vi "DeviceSelect.vi"() -> ()   [LabVIEW 2020]
uses:
  GlobalDeviceList.vi
panel:
  out "通道数量":string
  in  "全选按钮":T1
  in  "通道状态":cluster{"通道0":T2, "通道1":T2, "通道2":T2, "通道3":T2}
  out "勾选的设备":string[](array[string])
  in  "取消":T3
  in  "确定":T4
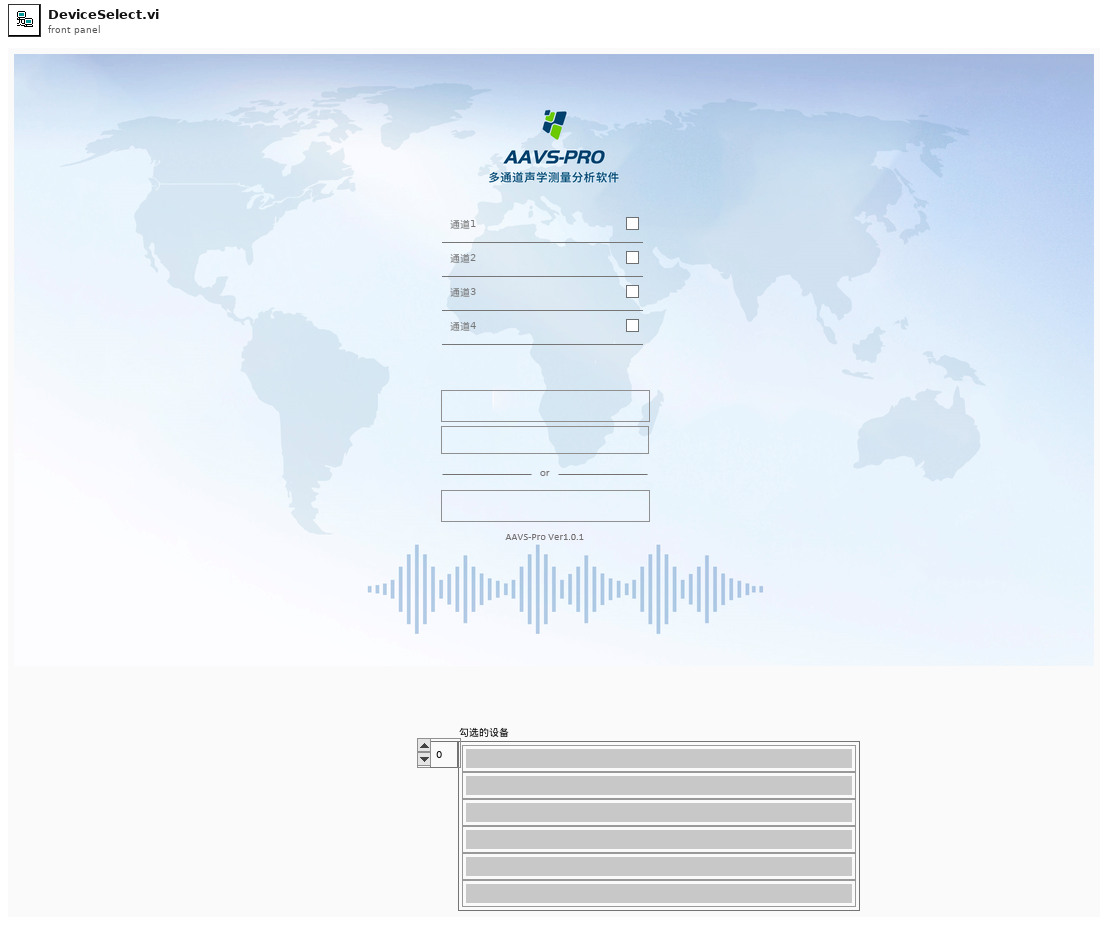
[diagram p1: front panel]
types:
  T1 = typedef "首页全选按钮.ctl" = bool
  T2 = typedef "首页复选框.ctl" = bool
  T3 = typedef "首页取消按钮.ctl" = bool
  T4 = typedef "首页确认按钮.ctl" = bool
  T5 = cluster{"通道0":bool, "通道1":bool, "通道2":bool, "通道3":bool}
  T6 = cluster{"勾选的设备":refnum<visa-resource-name>[], "设备启用状态":cluster{"通道0":bool, "通道1":bool, "通道2":bool, "通道3":bool}}
  T7 = enum32{"Invalid", "Standard", "Closed", "Hidden", "Minimized", "Maximized"}
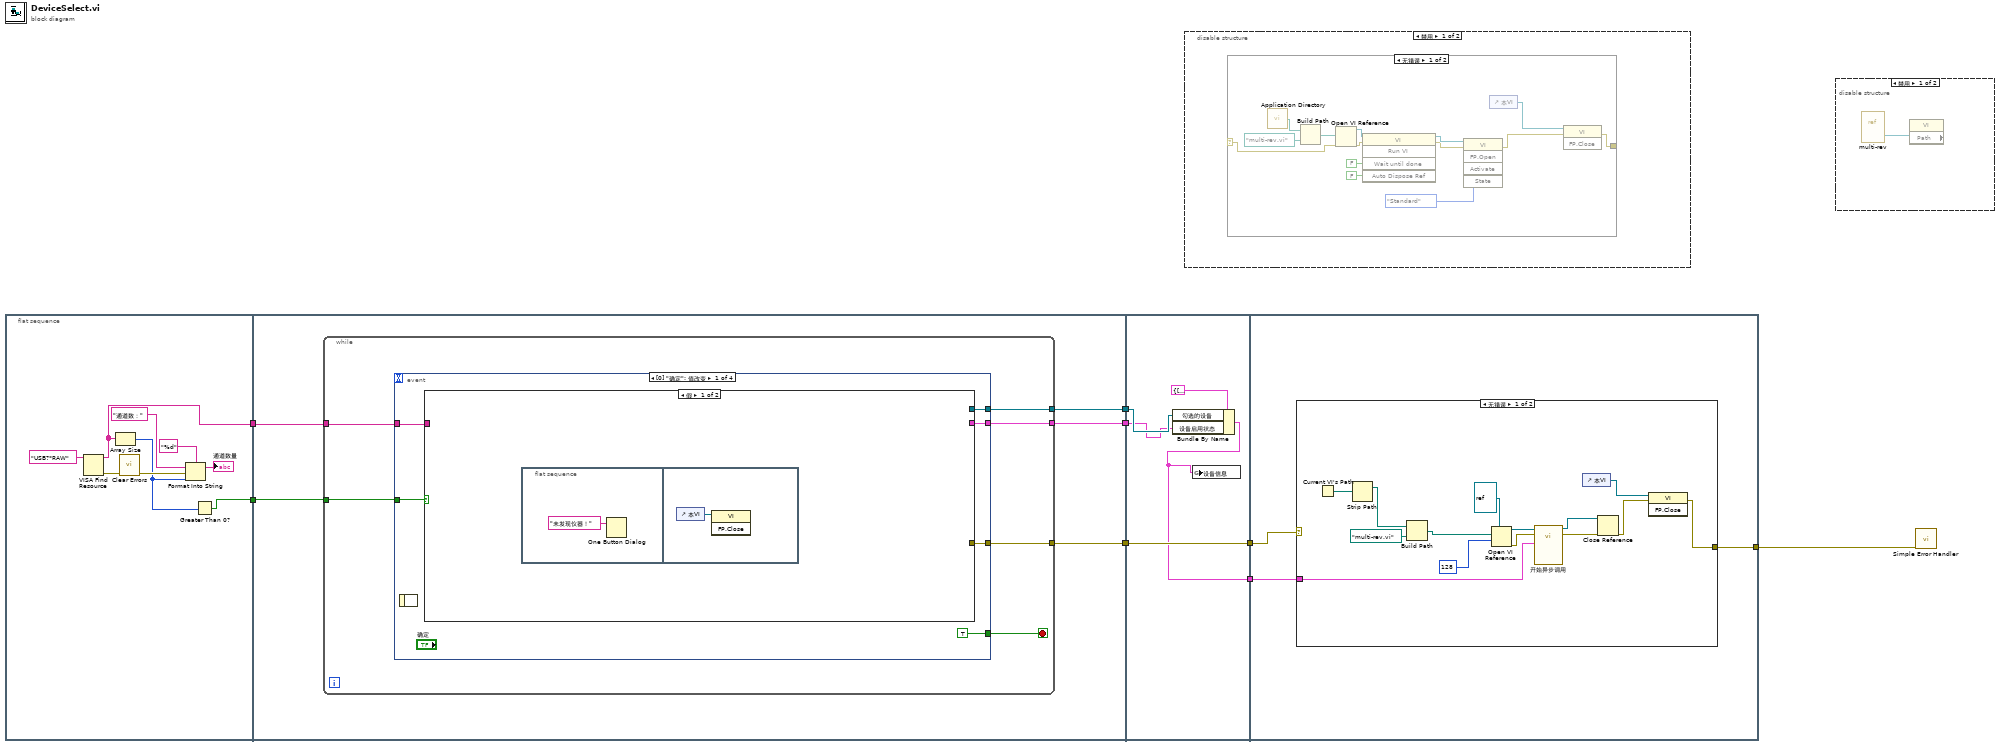
[diagram p0: block diagram]
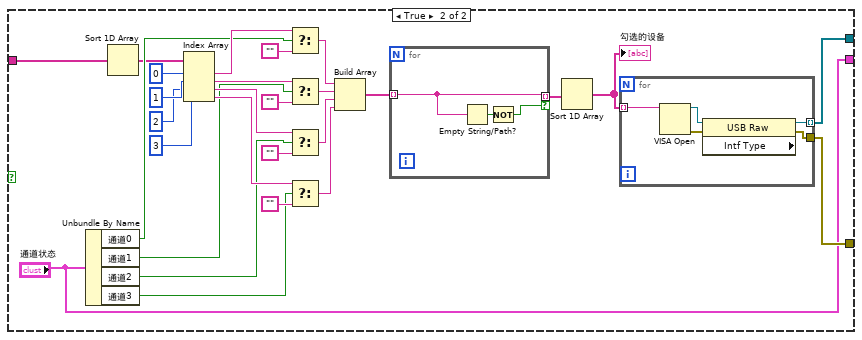
[diagram p5: hidden frame]
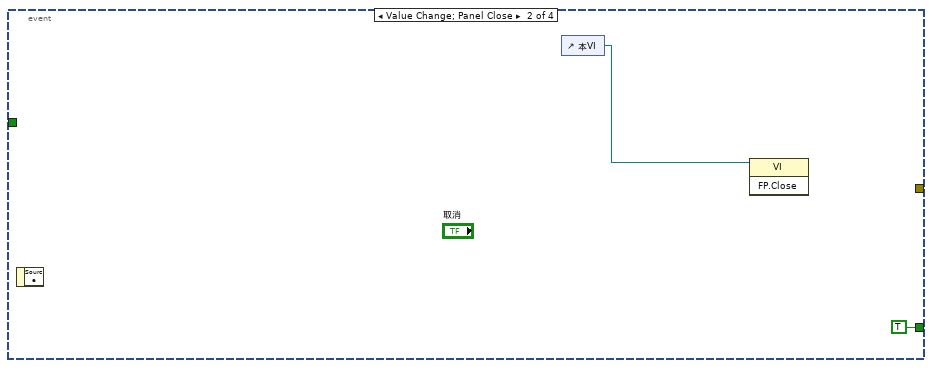
[diagram p6: hidden frame]
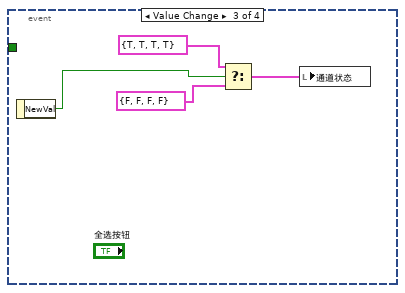
[diagram p7: hidden frame]
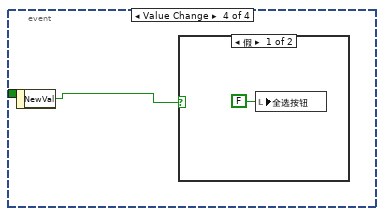
[diagram p8: hidden frame]
diagram:
  n1 = flat-sequence {
    tunnel: [w16] -> w2
    tunnel: [w9] -> w1
    tunnel: [w22] -> w7
    tunnel: [w21] -> w6
    tunnel: [w20] -> w4
    tunnel: w2 -> [w19]
    tunnel: w1 -> [w18]
    tunnel: w7 -> [w83]
    tunnel: w6 -> [w85]
    tunnel: [w85] -> w5
    tunnel: w4 -> [w82]
    tunnel: [w81] -> w3
    tunnel: [w86] -> w8
    tunnel: w5 -> [w88]
    tunnel: w3 -> [w87]
    frame #0 {
      n2 = VISA Find Resource(11:"USB?*RAW" ("表达式(\"?*\")")) -> (0:w12:errorcluster, 3:w16:string[])  [unwired: 2 in, 1 out]
      n3 = Array Size(array=w16) -> (size(s)=w10:i32)
      n4 = call <vilib>:"Clear Errors.vi"("error in (no error)"=w12) -> ("error out"=w11:errorcluster)  [unwired: 5 in, 1 out]
      n5 = Format Into String(format string="%d" ("格式字符串"), initial string="通道数：" ("初始字符串"), error in=w11, w10) -> (resulting string=→"通道数量":string)  [unwired: 1 out]
      n6 = Greater Than 0?(x=w10) -> (x > 0?=w9:bool)
    }
    frame #1 {
      n7 = while {
        tunnel: [w28] -> w22
        tunnel: [w27] -> w21
        tunnel: [w26] -> w20
        tunnel: w19 -> [w25]
        tunnel: w18 -> [w23]
        stop <- w24 stop-if-true
        n8 = event shown="[0] \"确定\": 值改变" {
          selector: _ -> [_ _ _ _]
          dyn-events: _ -> [_ _ _ _]
          timeout: _ -> [_ _ _ _]
          tunnel: [w34 _ _ _] -> w28
          tunnel: [w33 _ _ _] -> w27
          tunnel: [w31 _ _ _] -> w26
          tunnel: w25 -> [w32 _ _ _]
          tunnel: [TRUE TRUE _ _] -> w24
          tunnel: w23 -> [w29 _ _ _]
          event Value Change {
            n9 = event-data() -> ()  [unwired: 1 in, 1 out]
            n10 = case shown="假" w29 {
              tunnel: [_ w48] -> w34
              tunnel: [_ w47] -> w33
              tunnel: w32 -> [_ w41]
              tunnel: [_ "通道状态"] -> w31
              frame False {
                n11 = flat-sequence {
                  frame #0 {
                    n12 = One Button Dialog(message="未发现仪器！" ("消息")) -> ()  [unwired: 1 in, 1 out]
                  }
                  frame #1 {
                    n13 = control-ref of="本VI"() -> (w36:refnum<vi>)
                    n14 = invoke class="VI" method="FP.Close"(reference=w36) -> ()  [unwired: 2 in, 3 out]
                  }
                }
              }
              frame True {
                n15 = Unbundle By Name("通道状态") -> ("通道0"=w46:T2, "通道1"=w45:T2, "通道2"=w44:T2, "通道3"=w43:T2)
                n16 = Sort 1D Array(array=w41) -> (sorted array=w42:string[])
                n17 = Index Array(array=w42, index #1=0 ("索引"), index #2=1 ("索引"), index #3=2 ("索引"), index #4=3 ("索引")) -> (element #1=w57:string, element #2=w58:string, element #3=w59:string, element #4=w60:string)
                n18 = Select(t=w57, s=w46, f="") -> (s? t:f=w61:string)
                n19 = Select(t=w58, s=w45, f="") -> (s? t:f=w62:string)
                n20 = Select(t=w59, s=w44, f="") -> (s? t:f=w63:string)
                n21 = Select(t=w60, s=w43, f="") -> (s? t:f=w64:string)
                n22 = Build Array(w61, w62, w63, w64) -> (w39:string[])
                n23 = for {
                  tunnel: w39 -> [w67] mode=indexing
                  tunnel: [w67] -> w38 mode=indexing if=w65
                  n24 = Empty String/Path?(string/path=w67) -> (empty?=w66:bool)
                  n25 = Not(x=w66) -> (.not. x?=w65:bool)
                }
                n26 = Sort 1D Array(array=w38) -> (sorted array=w37:string[])
                "勾选的设备" <- w37
                n27 = for {
                  tunnel: w37 -> [w72] mode=indexing
                  tunnel: [w69] -> w48 mode=indexing
                  tunnel: [w68] -> w47
                  n28 = VISA Open(VISA resource name=w72) -> (VISA resource name=w71:refnum<visa-resource-name>, error out=w70:errorcluster)  [unwired: 4 in]
                  n29 = property class="USB Raw" props=["Intf Type"](reference=w71, error in=w70) -> (reference out=w69:refnum<visa-resource-name>, error out=w68:errorcluster)  [unwired: 1 out]
                }
              }
            }
          }
          event Value Change; Panel Close {
            n30 = event-data() -> ()  [unwired: 1 in, 1 out]
            n31 = control-ref of="本VI"() -> (w73:refnum<vi>)
            n32 = invoke class="VI" method="FP.Close"(reference=w73) -> ()  [unwired: 2 in, 3 out]
          }
          event Value Change {
            n33 = event-data() -> ("NewVal"=w78:T1)  [unwired: 1 in]
            n34 = Select(t=T5 {"通道0"=TRUE, "通道1"=TRUE, "通道2"=TRUE, "通道3"=TRUE} ("通道状态"), s=w78, f=T5 {"通道0"=FALSE, "通道1"=FALSE, "通道2"=FALSE, "通道3"=FALSE} ("通道状态")) -> (s? t:f=w75:T5)
            n35 = local write "通道状态"(w75) -> ()
          }
          event Value Change {
            n36 = event-data() -> ("NewVal"=w79:T2)  [unwired: 1 in]
            n37 = case shown="假" w79 {
              frame False {
                n38 = local write "全选按钮"(T1 FALSE ("全选按钮")) -> ()
              }
              frame True {
              }
            }
          }
        }
      }
    }
    frame #2 {
      n39 = Bundle By Name(cluster=T6 {"勾选的设备"=[], "设备启用状态"={"通道0"=FALSE, "通道1"=FALSE, "通道2"=FALSE, "通道3"=FALSE}} ("设备信息"), "勾选的设备"=w83, "设备启用状态"=w82) -> (w81:T6)
      n40 = global write "GlobalDeviceList.vi" "设备信息"(w81) -> ()
    }
    frame #3 {
      n41 = case shown="无错误" w88 {
        selector: w88 -> [_ w103]
        tunnel: w87 -> [w98 _]
        tunnel: [w93 w103] -> w86
        frame No Error {
          n42 = Current VI's Path() -> (path=w91:path)
          n43 = Strip Path(path=w91) -> (stripped path=w92:path)  [unwired: 1 out]
          n44 = Build Path(base path=w92, name or relative path=path "multi-rev.vi" ("名称或相对路径")) -> (appended path=w89:path)
          n45 = Open VI Reference(type specifier VI Refnum (for type only)=refnum<vi> refnum ("类型说明符VI引用句柄（仅用于类型）"), vi path=w89, options=128 ("选项")) -> (vi reference=w100:refnum<vi>, error out=w99:errorcluster)  [unwired: 3 in]
          n46 = call-by-ref "开始异步调用"(reference=w100, error in=w99, "设备信息"=w98) -> (reference out=w96:refnum<vi>, error out=w97:errorcluster)  [unwired: 11 in]
          n47 = control-ref of="本VI"() -> (w95:refnum<vi>)
          n48 = Close Reference(reference=w96, error in (no error)=w97) -> (error out=w94:errorcluster)
          n49 = invoke class="VI" method="FP.Close"(reference=w95, error in=w94) -> (error out=w93:errorcluster)  [unwired: 1 in, 2 out]
        }
        frame Error {
        }
      }
    }
  }
  n50 = disable-structure shown="禁用" {
    frame Disabled {
      n51 = case shown="无错误" {
        selector: _ -> [w104 w118]
        tunnel: [w105 w118] -> _
        frame No Error {
          n52 = call <vilib>:"Application Directory.vi"() -> ("Application Directory"=w115:path)
          n53 = Build Path(base path=w115, name or relative path=path "multi-rev.vi" ("名称或相对路径")) -> (appended path=w116:path)
          n54 = Open VI Reference(vi path=w116, error in (no error)=w104) -> (vi reference=w113:refnum<vi>, error out=w108:errorcluster)  [unwired: 4 in]
          n55 = invoke class="VI" method="Run VI"(reference=w113, error in=w108, "Wait until done"=FALSE ("结束前等待"), "Auto Dispose Ref"=FALSE ("自动销毁引用")) -> (reference out=w110:refnum<vi>, error out=w107:errorcluster)  [unwired: 1 in, 3 out]
          n56 = invoke class="VI" method="FP.Open"(reference=w110, error in=w107, "State"=T7."Standard" ("状态")) -> (error out=w106:errorcluster)  [unwired: 2 in, 4 out]
          n57 = control-ref of="本VI"() -> (w117:refnum<vi>)
          n58 = invoke class="VI" method="FP.Close"(reference=w117, error in=w106) -> (error out=w105:errorcluster)  [unwired: 1 in, 2 out]
        }
        frame Error {
        }
      }
    }
    frame Enabled {
    }
  }
  n59 = disable-structure shown="禁用" {
    frame Disabled {
      n60 = vi-ref "multi-rev.vi"() -> (w119:refnum<vi>)
      n61 = property class="VI" props=["Path"](reference=w119) -> ()  [unwired: 1 in, 3 out]
    }
    frame Enabled {
    }
  }
  n62 = call <vilib>:"Simple Error Handler.vi"("error in (no error)"=w8) -> ()  [unwired: 4 in, 5 out]
